vi "XML ( Save ).vi"(8 "error in (no error)":errorcluster, 10 "Path":path, 11 "XML in":refnum<class "XML.lvclass">) -> (0 "error out":errorcluster, 3 "XML out":refnum<class "XML.lvclass">)   [LabVIEW 2018, in "XML.lvlib" / "XML.lvclass"]
uses:
  XML.lvclass
  XML.lvclass/XML.ctl
  <vilib>/xml/Close Reference(Node).vi
  <vilib>/xml/NI_XML.lvlib
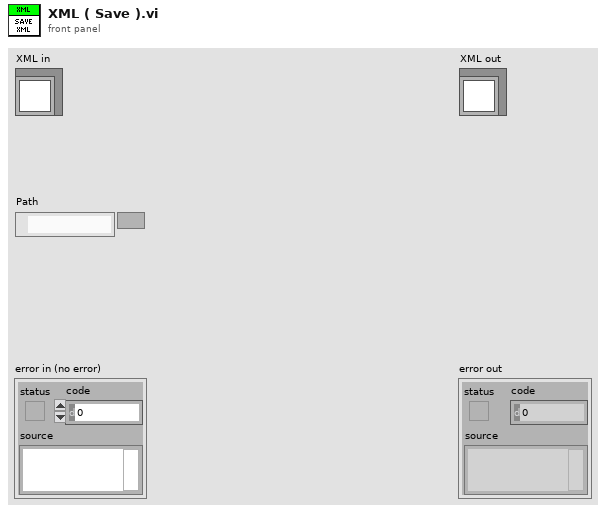
[diagram p1: front panel]
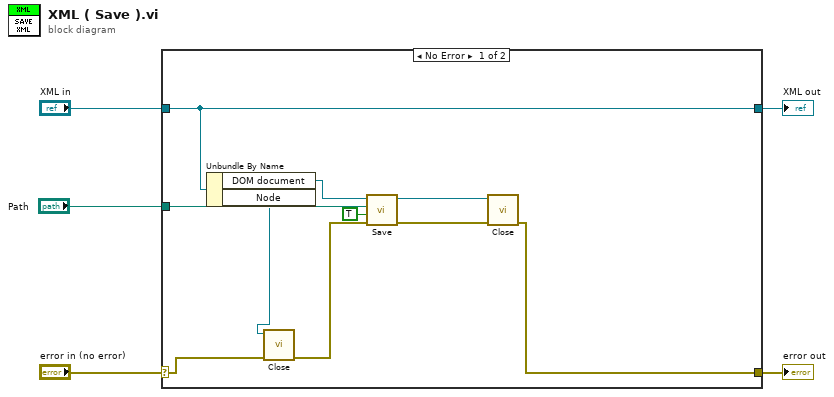
[diagram p0: block diagram]
diagram:
  n1 = case shown="No Error" "error in (no error)" {
    selector: "error in (no error)" -> [w8 w17]
    tunnel: [w13 w17] -> w4
    tunnel: [w12 w16] -> w2
    tunnel: "XML in" -> [w12 w16]
    tunnel: "Path" -> [w10 _]
    frame No Error {
      n2 = Unbundle By Name(w12) -> ("DOM document"=w11:refnum<k20>, "Node"=w6:refnum<k20>)
      n3 = call-poly <vilib>:"Close.vi"("error in (no error)"=w8, "node"=w6) -> ("error out"=w7:errorcluster)  [unwired: 7 in]
      n4 = call <vilib>:"Save.vi"("error in (no error)"=w7, "overwrite file (True)"=TRUE, "XML file path"=w10, "DOM document in"=w11) -> ("error out"=w15:errorcluster, "DOM document out"=w14:refnum<k20>)  [unwired: 5 in, 1 out]
      n5 = call-poly <vilib>:"Close.vi"("error in (no error)"=w15, "node"=w14) -> ("error out"=w13:errorcluster)  [unwired: 7 in]
    }
    frame Error {
    }
  }
  "error out" <- w4
  "XML out" <- w2
